vi "SVT UFF58 Get Function References.vi"(0 "file refnum":refnum<k20>, 5 "function type (all functions:0)":T2, 11 "error in (no error)":errorcluster) -> (4 "dup file refnum":refnum<k20>, 6 "function refnums":refnum<k20>[](array[refnum]), 8 "function types":T1[](array[typedef]), 10 "number of functions":i32, 15 "error out":errorcluster)   [LabVIEW 2017, in "SoundVib_UFF58.lvlib"]
doc: "Retrieves the function references and the function types of all the functions specified by <B>function type</B> that are present in the UFF58 (universal file format) file specified by <B>file refnum</B>."
uses:
  <vilib>/addons/Sound and Vibration/svt_UFF58/SoundVib_UFF58.lvlib
  <vilib>/addons/Sound and Vibration/svt_UFF58/subVIs/sv_UFF58 Get FunctionType.ctl
  <vilib>/addons/Sound and Vibration/svt_UFF58/subVIs/sv_FunctionType.ctl
  <vilib>/Platform/storage/Storage.llb/Get Property (Storage Refnums).vi
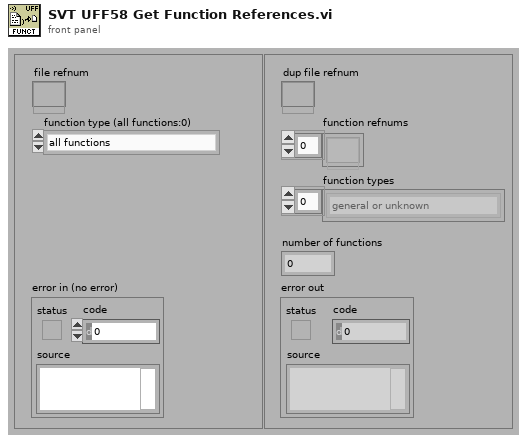
[diagram p1: front panel]
types:
  T1 = typedef "SoundVib_UFF58.lvlib/sv_FunctionType.ctl" = enum16{"general or unknown", "time response", "auto spectrum", "cross spectrum", "frequency response function", "transmissibility", "coherence", "auto correlation", "cross correlation", "power spectral density (PSD)", "energy spectral density (ESD)", "probability density function", "spectrum", "cumulative frequency distribution", "peaks valley", "stress/cycles", "strain/cycles", "orbit", "mode indicator function", "force pattern", "partial power", "partial coherence", "eigenvalue", "eigenvector", "shock response spectrum", "finite impulse response filter", "multiple coherence", "order function", "phase compensation"}
  T2 = typedef "SoundVib_UFF58.lvlib/sv_UFF58 Get FunctionType.ctl" = enum16{"all functions", "all time waveforms", "all spectra (real)", "all spectra (complex)", "general or unknown", "time response", "auto spectrum", "cross spectrum", "frequency response function", "transmissibility", "coherence", "auto correlation", "cross correlation", "power spectral density (PSD)", "energy spectral density (ESD)", "probability density function", "spectrum", "cumulative frequency distribution", "peaks valley", "stress/cycles", "strain/cycles", "orbit", "mode indicator function", "force pattern", "partial power", "partial coherence", "eigenvalue", "eigenvector", "shock response spectrum", "finite impulse response filter", "multiple coherence", "order function"}
  T3 = typedef "SoundVib_UFF58.lvlib/sv_UFF58 DOF.ctl" = cluster{"function type":T1, "function ID number":i32, "version number":i32, "load case ID number":i32, "response entity name":string, "response node":i32, "response direction":T4, "reference entity name":string, "reference node":i32, "reference direction":T4}
  T4 = typedef "SoundVib_UFF58.lvlib/sv_UFF58 Response Direction.ctl" = i32
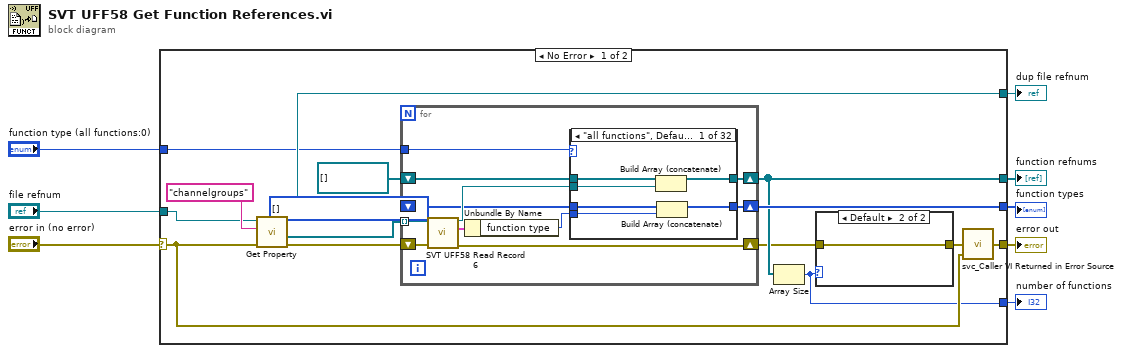
[diagram p0: block diagram]
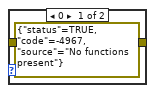
[diagram p2: hidden frame]
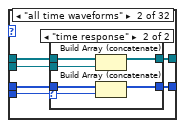
[diagram p3: hidden frame]
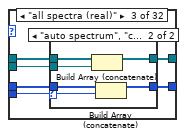
[diagram p5: hidden frame]
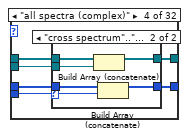
[diagram p7: hidden frame]
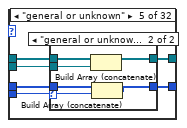
[diagram p9: hidden frame]
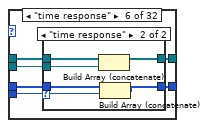
[diagram p11: hidden frame]
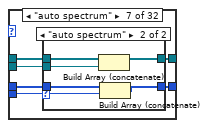
[diagram p13: hidden frame]
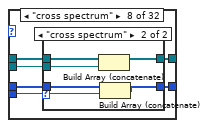
[diagram p15: hidden frame]
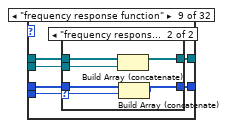
[diagram p17: hidden frame]
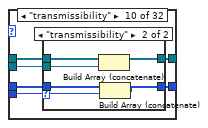
[diagram p19: hidden frame]
diagram:
  n1 = case shown="No Error" "error in (no error)" {
    selector: "error in (no error)" -> [w18 w477]
    tunnel: "file refnum" -> [w22 w478]
    tunnel: [w21 w478] -> w2
    tunnel: [w11 _] -> w7
    tunnel: [w12 _] -> w6
    tunnel: [w14 _] -> w5
    tunnel: [w19 w477] -> w4
    tunnel: "function type (all functions:0)" -> [w15 _]
    frame No Error {
      w16 = T1[] [] items=["general or unknown", "time response", "auto spectrum", "cross spectrum", "frequency response function", "transmissibility", "coherence", "auto correlation", "cross correlation", "power spectral density (PSD)", "energy spectral density (ESD)", "probability density function", "spectrum", "cumulative frequency distribution", "peaks valley", "stress/cycles", "strain/cycles", "orbit", "mode indicator function", "force pattern", "partial power", "partial coherence", "eigenvalue", "eigenvector", "shock response spectrum", "finite impulse response filter", "multiple coherence", "order function", "phase compensation"]
      n2 = call-poly <vilib>:"Get Property.vi"("error in (no error)"=w18, "Property name"="channelgroups", "storage refnum"=w22) -> ("error out"=w20:errorcluster, "Value"=w17:refnum<k20>[], "storage refnum out"=w21:refnum<k20>)  [unwired: 6 in]
      n3 = for {
        tunnel: w17 -> [w33] mode=indexing
        shift-right: [w34] -> w10
        shift-left: w20 -> [w35]
        shift-right: [w26] -> w12
        shift-left: refnum<k20>[] [] -> [w27]
        tunnel: w15 -> [w32]
        shift-right: [w30] -> w14
        shift-left: w16 -> [w28]
        n4 = call <vilib>:"SVT UFF58 Read Record 6.vi"("function refnum"=w33, "error in (no error)"=w35) -> ("dup function refnum"=w29:refnum<k20>, "DOF identification"=w36:T3, "error out"=w34:errorcluster)  [unwired: 11 in]
        n5 = Unbundle By Name(w36) -> ("function type"=w31:T1)
        n6 = case shown="\"all functions\", Default" w32 {
          tunnel: w31 -> [w41 w46 w62 w76 w89 w103 w117 w131 w145 w159 w173 w187 w201 w215 w229 w243 w257 w271 w285 w299 w313 w327 w341 w355 w369 w383 w397 w411 w425 w439 w453 w467]
          tunnel: w28 -> [w42 w48 w61 w75 w90 w104 w118 w132 w146 w160 w174 w188 w202 w216 w230 w244 w258 w272 w286 w300 w314 w328 w342 w356 w370 w384 w398 w412 w426 w440 w454 w468]
          tunnel: [w40 w47 w60 w74 w88 w102 w116 w130 w144 w158 w172 w186 w200 w214 w228 w242 w256 w270 w284 w298 w312 w326 w340 w354 w368 w382 w396 w410 w424 w438 w452 w466] -> w30
          tunnel: w29 -> [w38 w44 w58 w72 w85 w99 w113 w127 w141 w155 w169 w183 w197 w211 w225 w239 w253 w267 w281 w295 w309 w323 w337 w351 w365 w379 w393 w407 w421 w435 w449 w463]
          tunnel: w27 -> [w39 w45 w59 w73 w87 w101 w115 w129 w143 w157 w171 w185 w199 w213 w227 w241 w255 w269 w283 w297 w311 w325 w339 w353 w367 w381 w395 w409 w423 w437 w451 w465]
          tunnel: [w37 w43 w57 w71 w86 w100 w114 w128 w142 w156 w170 w184 w198 w212 w226 w240 w254 w268 w282 w296 w310 w324 w338 w352 w366 w380 w394 w408 w422 w436 w450 w464] -> w26
          frame "all functions", Default {
            n7 = Build Array (concatenate)(w39, w38) -> (w37:refnum<k20>[])
            n8 = Build Array (concatenate)(w42, w41) -> (w40:T1[])
          }
          frame "all time waveforms" {
            n9 = case shown="\"time response\"" w46 {
              selector: w46 -> [_ w54]
              tunnel: w48 -> [w50 w56]
              tunnel: [w50 w55] -> w47
              tunnel: w45 -> [w49 w53]
              tunnel: w44 -> [_ w52]
              tunnel: [w49 w51] -> w43
              frame Default {
              }
              frame "time response" {
                n10 = Build Array (concatenate)(w53, w52) -> (w51:refnum<k20>[])
                n11 = Build Array (concatenate)(w56, w54) -> (w55:T1[])
              }
            }
          }
          frame "all spectra (real)" {
            n12 = case shown="\"auto spectrum\", \"coherence\", \"power spectral density (PSD)\", \"energy spectral density (ESD)\", \"spectrum\", \"partial power\", \"partial coherence\", \"shock response spectrum\"" w62 {
              selector: w62 -> [_ w68]
              tunnel: w61 -> [w64 w70]
              tunnel: [w64 w69] -> w60
              tunnel: w59 -> [w63 w67]
              tunnel: w58 -> [_ w66]
              tunnel: [w63 w65] -> w57
              frame Default {
              }
              frame "auto spectrum", "coherence", "power spectral density (PSD)", "energy spectral density (ESD)", "spectrum", "partial power", "partial coherence", "shock response spectrum" {
                n13 = Build Array (concatenate)(w67, w66) -> (w65:refnum<k20>[])
                n14 = Build Array (concatenate)(w70, w68) -> (w69:T1[])
              }
            }
          }
          frame "all spectra (complex)" {
            n15 = case shown="\"cross spectrum\"..\"transmissibility\", \"peaks valley\"..\"orbit\"" w76 {
              selector: w76 -> [_ w82]
              tunnel: w75 -> [w78 w84]
              tunnel: [w78 w83] -> w74
              tunnel: w73 -> [w77 w81]
              tunnel: w72 -> [_ w80]
              tunnel: [w77 w79] -> w71
              frame Default {
              }
              frame "cross spectrum".."transmissibility", "peaks valley".."orbit" {
                n16 = Build Array (concatenate)(w81, w80) -> (w79:refnum<k20>[])
                n17 = Build Array (concatenate)(w84, w82) -> (w83:T1[])
              }
            }
          }
          frame "general or unknown" {
            n18 = case shown="\"general or unknown\"" w89 {
              selector: w89 -> [_ w97]
              tunnel: w90 -> [w92 w98]
              tunnel: [w92 w96] -> w88
              tunnel: w87 -> [w91 w95]
              tunnel: [w91 w94] -> w86
              tunnel: w85 -> [_ w93]
              frame Default {
              }
              frame "general or unknown" {
                n19 = Build Array (concatenate)(w95, w93) -> (w94:refnum<k20>[])
                n20 = Build Array (concatenate)(w98, w97) -> (w96:T1[])
              }
            }
          }
          frame "time response" {
            n21 = case shown="\"time response\"" w103 {
              selector: w103 -> [_ w111]
              tunnel: w104 -> [w106 w112]
              tunnel: [w106 w110] -> w102
              tunnel: w101 -> [w105 w109]
              tunnel: [w105 w108] -> w100
              tunnel: w99 -> [_ w107]
              frame Default {
              }
              frame "time response" {
                n22 = Build Array (concatenate)(w109, w107) -> (w108:refnum<k20>[])
                n23 = Build Array (concatenate)(w112, w111) -> (w110:T1[])
              }
            }
          }
          frame "auto spectrum" {
            n24 = case shown="\"auto spectrum\"" w117 {
              selector: w117 -> [_ w125]
              tunnel: w118 -> [w120 w126]
              tunnel: [w120 w124] -> w116
              tunnel: w115 -> [w119 w123]
              tunnel: [w119 w122] -> w114
              tunnel: w113 -> [_ w121]
              frame Default {
              }
              frame "auto spectrum" {
                n25 = Build Array (concatenate)(w123, w121) -> (w122:refnum<k20>[])
                n26 = Build Array (concatenate)(w126, w125) -> (w124:T1[])
              }
            }
          }
          frame "cross spectrum" {
            n27 = case shown="\"cross spectrum\"" w131 {
              selector: w131 -> [_ w139]
              tunnel: w132 -> [w134 w140]
              tunnel: [w134 w138] -> w130
              tunnel: w129 -> [w133 w137]
              tunnel: [w133 w136] -> w128
              tunnel: w127 -> [_ w135]
              frame Default {
              }
              frame "cross spectrum" {
                n28 = Build Array (concatenate)(w137, w135) -> (w136:refnum<k20>[])
                n29 = Build Array (concatenate)(w140, w139) -> (w138:T1[])
              }
            }
          }
          frame "frequency response function" {
            n30 = case shown="\"frequency response function\"" w145 {
              selector: w145 -> [_ w153]
              tunnel: w146 -> [w148 w154]
              tunnel: [w148 w152] -> w144
              tunnel: w143 -> [w147 w151]
              tunnel: [w147 w150] -> w142
              tunnel: w141 -> [_ w149]
              frame Default {
              }
              frame "frequency response function" {
                n31 = Build Array (concatenate)(w151, w149) -> (w150:refnum<k20>[])
                n32 = Build Array (concatenate)(w154, w153) -> (w152:T1[])
              }
            }
          }
          frame "transmissibility" {
            n33 = case shown="\"transmissibility\"" w159 {
              selector: w159 -> [_ w167]
              tunnel: w160 -> [w162 w168]
              tunnel: [w162 w166] -> w158
              tunnel: w157 -> [w161 w165]
              tunnel: [w161 w164] -> w156
              tunnel: w155 -> [_ w163]
              frame Default {
              }
              frame "transmissibility" {
                n34 = Build Array (concatenate)(w165, w163) -> (w164:refnum<k20>[])
                n35 = Build Array (concatenate)(w168, w167) -> (w166:T1[])
              }
            }
          }
          frame "coherence" {
            n36 = case shown="\"coherence\"" w173 {
              selector: w173 -> [_ w181]
              tunnel: w174 -> [w176 w182]
              tunnel: [w176 w180] -> w172
              tunnel: w171 -> [w175 w179]
              tunnel: [w175 w178] -> w170
              tunnel: w169 -> [_ w177]
              frame Default {
              }
              frame "coherence" {
                n37 = Build Array (concatenate)(w179, w177) -> (w178:refnum<k20>[])
                n38 = Build Array (concatenate)(w182, w181) -> (w180:T1[])
              }
            }
          }
          frame "auto correlation" {
            n39 = case shown="\"auto correlation\"" w187 {
              selector: w187 -> [_ w195]
              tunnel: w188 -> [w190 w196]
              tunnel: [w190 w194] -> w186
              tunnel: w185 -> [w189 w193]
              tunnel: [w189 w192] -> w184
              tunnel: w183 -> [_ w191]
              frame Default {
              }
              frame "auto correlation" {
                n40 = Build Array (concatenate)(w193, w191) -> (w192:refnum<k20>[])
                n41 = Build Array (concatenate)(w196, w195) -> (w194:T1[])
              }
            }
          }
          frame "cross correlation" {
            n42 = case shown="\"cross correlation\"" w201 {
              selector: w201 -> [_ w209]
              tunnel: w202 -> [w204 w210]
              tunnel: [w204 w208] -> w200
              tunnel: w199 -> [w203 w207]
              tunnel: [w203 w206] -> w198
              tunnel: w197 -> [_ w205]
              frame Default {
              }
              frame "cross correlation" {
                n43 = Build Array (concatenate)(w207, w205) -> (w206:refnum<k20>[])
                n44 = Build Array (concatenate)(w210, w209) -> (w208:T1[])
              }
            }
          }
          frame "power spectral density (PSD)" {
            n45 = case shown="\"power spectral density (PSD)\"" w215 {
              selector: w215 -> [_ w223]
              tunnel: w216 -> [w218 w224]
              tunnel: [w218 w222] -> w214
              tunnel: w213 -> [w217 w221]
              tunnel: [w217 w220] -> w212
              tunnel: w211 -> [_ w219]
              frame Default {
              }
              frame "power spectral density (PSD)" {
                n46 = Build Array (concatenate)(w221, w219) -> (w220:refnum<k20>[])
                n47 = Build Array (concatenate)(w224, w223) -> (w222:T1[])
              }
            }
          }
          frame "energy spectral density (ESD)" {
            n48 = case shown="\"energy spectral density (ESD)\"" w229 {
              selector: w229 -> [_ w237]
              tunnel: w230 -> [w232 w238]
              tunnel: [w232 w236] -> w228
              tunnel: w227 -> [w231 w235]
              tunnel: [w231 w234] -> w226
              tunnel: w225 -> [_ w233]
              frame Default {
              }
              frame "energy spectral density (ESD)" {
                n49 = Build Array (concatenate)(w235, w233) -> (w234:refnum<k20>[])
                n50 = Build Array (concatenate)(w238, w237) -> (w236:T1[])
              }
            }
          }
          frame "probability density function" {
            n51 = case shown="\"probability density function\"" w243 {
              selector: w243 -> [_ w251]
              tunnel: w244 -> [w246 w252]
              tunnel: [w246 w250] -> w242
              tunnel: w241 -> [w245 w249]
              tunnel: [w245 w248] -> w240
              tunnel: w239 -> [_ w247]
              frame Default {
              }
              frame "probability density function" {
                n52 = Build Array (concatenate)(w249, w247) -> (w248:refnum<k20>[])
                n53 = Build Array (concatenate)(w252, w251) -> (w250:T1[])
              }
            }
          }
          frame "spectrum" {
            n54 = case shown="\"spectrum\"" w257 {
              selector: w257 -> [_ w265]
              tunnel: w258 -> [w260 w266]
              tunnel: [w260 w264] -> w256
              tunnel: w255 -> [w259 w263]
              tunnel: [w259 w262] -> w254
              tunnel: w253 -> [_ w261]
              frame Default {
              }
              frame "spectrum" {
                n55 = Build Array (concatenate)(w263, w261) -> (w262:refnum<k20>[])
                n56 = Build Array (concatenate)(w266, w265) -> (w264:T1[])
              }
            }
          }
          frame "cumulative frequency distribution" {
            n57 = case shown="\"cumulative frequency distribution\"" w271 {
              selector: w271 -> [_ w279]
              tunnel: w272 -> [w274 w280]
              tunnel: [w274 w278] -> w270
              tunnel: w269 -> [w273 w277]
              tunnel: [w273 w276] -> w268
              tunnel: w267 -> [_ w275]
              frame Default {
              }
              frame "cumulative frequency distribution" {
                n58 = Build Array (concatenate)(w277, w275) -> (w276:refnum<k20>[])
                n59 = Build Array (concatenate)(w280, w279) -> (w278:T1[])
              }
            }
          }
          frame "peaks valley" {
            n60 = case shown="\"peaks valley\"" w285 {
              selector: w285 -> [_ w293]
              tunnel: w286 -> [w288 w294]
              tunnel: [w288 w292] -> w284
              tunnel: w283 -> [w287 w291]
              tunnel: [w287 w290] -> w282
              tunnel: w281 -> [_ w289]
              frame Default {
              }
              frame "peaks valley" {
                n61 = Build Array (concatenate)(w291, w289) -> (w290:refnum<k20>[])
                n62 = Build Array (concatenate)(w294, w293) -> (w292:T1[])
              }
            }
          }
          frame "stress/cycles" {
            n63 = case shown="\"stress/cycles\"" w299 {
              selector: w299 -> [_ w307]
              tunnel: w300 -> [w302 w308]
              tunnel: [w302 w306] -> w298
              tunnel: w297 -> [w301 w305]
              tunnel: [w301 w304] -> w296
              tunnel: w295 -> [_ w303]
              frame Default {
              }
              frame "stress/cycles" {
                n64 = Build Array (concatenate)(w305, w303) -> (w304:refnum<k20>[])
                n65 = Build Array (concatenate)(w308, w307) -> (w306:T1[])
              }
            }
          }
          frame "strain/cycles" {
            n66 = case shown="\"strain/cycles\"" w313 {
              selector: w313 -> [_ w321]
              tunnel: w314 -> [w316 w322]
              tunnel: [w316 w320] -> w312
              tunnel: w311 -> [w315 w319]
              tunnel: [w315 w318] -> w310
              tunnel: w309 -> [_ w317]
              frame Default {
              }
              frame "strain/cycles" {
                n67 = Build Array (concatenate)(w319, w317) -> (w318:refnum<k20>[])
                n68 = Build Array (concatenate)(w322, w321) -> (w320:T1[])
              }
            }
          }
          frame "orbit" {
            n69 = case shown="\"orbit\"" w327 {
              selector: w327 -> [_ w335]
              tunnel: w328 -> [w330 w336]
              tunnel: [w330 w334] -> w326
              tunnel: w325 -> [w329 w333]
              tunnel: [w329 w332] -> w324
              tunnel: w323 -> [_ w331]
              frame Default {
              }
              frame "orbit" {
                n70 = Build Array (concatenate)(w333, w331) -> (w332:refnum<k20>[])
                n71 = Build Array (concatenate)(w336, w335) -> (w334:T1[])
              }
            }
          }
          frame "mode indicator function" {
            n72 = case shown="\"mode indicator function\"" w341 {
              selector: w341 -> [_ w349]
              tunnel: w342 -> [w344 w350]
              tunnel: [w344 w348] -> w340
              tunnel: w339 -> [w343 w347]
              tunnel: [w343 w346] -> w338
              tunnel: w337 -> [_ w345]
              frame Default {
              }
              frame "mode indicator function" {
                n73 = Build Array (concatenate)(w347, w345) -> (w346:refnum<k20>[])
                n74 = Build Array (concatenate)(w350, w349) -> (w348:T1[])
              }
            }
          }
          frame "force pattern" {
            n75 = case shown="\"force pattern\"" w355 {
              selector: w355 -> [_ w363]
              tunnel: w356 -> [w358 w364]
              tunnel: [w358 w362] -> w354
              tunnel: w353 -> [w357 w361]
              tunnel: [w357 w360] -> w352
              tunnel: w351 -> [_ w359]
              frame Default {
              }
              frame "force pattern" {
                n76 = Build Array (concatenate)(w361, w359) -> (w360:refnum<k20>[])
                n77 = Build Array (concatenate)(w364, w363) -> (w362:T1[])
              }
            }
          }
          frame "partial power" {
            n78 = case shown="\"partial power\"" w369 {
              selector: w369 -> [_ w377]
              tunnel: w370 -> [w372 w378]
              tunnel: [w372 w376] -> w368
              tunnel: w367 -> [w371 w375]
              tunnel: [w371 w374] -> w366
              tunnel: w365 -> [_ w373]
              frame Default {
              }
              frame "partial power" {
                n79 = Build Array (concatenate)(w375, w373) -> (w374:refnum<k20>[])
                n80 = Build Array (concatenate)(w378, w377) -> (w376:T1[])
              }
            }
          }
          frame "partial coherence" {
            n81 = case shown="\"partial coherence\"" w383 {
              selector: w383 -> [_ w391]
              tunnel: w384 -> [w386 w392]
              tunnel: [w386 w390] -> w382
              tunnel: w381 -> [w385 w389]
              tunnel: [w385 w388] -> w380
              tunnel: w379 -> [_ w387]
              frame Default {
              }
              frame "partial coherence" {
                n82 = Build Array (concatenate)(w389, w387) -> (w388:refnum<k20>[])
                n83 = Build Array (concatenate)(w392, w391) -> (w390:T1[])
              }
            }
          }
          frame "eigenvalue" {
            n84 = case shown="\"eigenvalue\"" w397 {
              selector: w397 -> [_ w405]
              tunnel: w398 -> [w400 w406]
              tunnel: [w400 w404] -> w396
              tunnel: w395 -> [w399 w403]
              tunnel: [w399 w402] -> w394
              tunnel: w393 -> [_ w401]
              frame Default {
              }
              frame "eigenvalue" {
                n85 = Build Array (concatenate)(w403, w401) -> (w402:refnum<k20>[])
                n86 = Build Array (concatenate)(w406, w405) -> (w404:T1[])
              }
            }
          }
          frame "eigenvector" {
            n87 = case shown="\"eigenvector\"" w411 {
              selector: w411 -> [_ w419]
              tunnel: w412 -> [w414 w420]
              tunnel: [w414 w418] -> w410
              tunnel: w409 -> [w413 w417]
              tunnel: [w413 w416] -> w408
              tunnel: w407 -> [_ w415]
              frame Default {
              }
              frame "eigenvector" {
                n88 = Build Array (concatenate)(w417, w415) -> (w416:refnum<k20>[])
                n89 = Build Array (concatenate)(w420, w419) -> (w418:T1[])
              }
            }
          }
          frame "shock response spectrum" {
            n90 = case shown="\"shock response spectrum\"" w425 {
              selector: w425 -> [_ w433]
              tunnel: w426 -> [w428 w434]
              tunnel: [w428 w432] -> w424
              tunnel: w423 -> [w427 w431]
              tunnel: [w427 w430] -> w422
              tunnel: w421 -> [_ w429]
              frame Default {
              }
              frame "shock response spectrum" {
                n91 = Build Array (concatenate)(w431, w429) -> (w430:refnum<k20>[])
                n92 = Build Array (concatenate)(w434, w433) -> (w432:T1[])
              }
            }
          }
          frame "finite impulse response filter" {
            n93 = case shown="\"finite impulse response filter\"" w439 {
              selector: w439 -> [_ w447]
              tunnel: w440 -> [w442 w448]
              tunnel: [w442 w446] -> w438
              tunnel: w437 -> [w441 w445]
              tunnel: [w441 w444] -> w436
              tunnel: w435 -> [_ w443]
              frame Default {
              }
              frame "finite impulse response filter" {
                n94 = Build Array (concatenate)(w445, w443) -> (w444:refnum<k20>[])
                n95 = Build Array (concatenate)(w448, w447) -> (w446:T1[])
              }
            }
          }
          frame "multiple coherence" {
            n96 = case shown="\"multiple coherence\"" w453 {
              selector: w453 -> [_ w461]
              tunnel: w454 -> [w456 w462]
              tunnel: [w456 w460] -> w452
              tunnel: w451 -> [w455 w459]
              tunnel: [w455 w458] -> w450
              tunnel: w449 -> [_ w457]
              frame Default {
              }
              frame "multiple coherence" {
                n97 = Build Array (concatenate)(w459, w457) -> (w458:refnum<k20>[])
                n98 = Build Array (concatenate)(w462, w461) -> (w460:T1[])
              }
            }
          }
          frame "order function" {
            n99 = case shown="\"order function\"" w467 {
              selector: w467 -> [_ w475]
              tunnel: w468 -> [w470 w476]
              tunnel: [w470 w474] -> w466
              tunnel: w465 -> [w469 w473]
              tunnel: [w469 w472] -> w464
              tunnel: w463 -> [_ w471]
              frame Default {
              }
              frame "order function" {
                n100 = Build Array (concatenate)(w473, w471) -> (w472:refnum<k20>[])
                n101 = Build Array (concatenate)(w476, w475) -> (w474:T1[])
              }
            }
          }
        }
      }
      n102 = Array Size(array=w12) -> (size(s)=w11:i32)
      n103 = case shown="Default" w11 {
        tunnel: w10 -> [_ w25]
        tunnel: [errorcluster {"status"=TRUE, "code"=-4967, "source"="No functions present"} ("error out") w25] -> w9
        frame 0 {
        }
        frame Default {
        }
      }
      n104 = call <vilib>:"svc_Caller VI Returned in Error Source.vi"("warning input to caller"=w18, "error in (no error)"=w9) -> ("error out"=w19:errorcluster)  [unwired: 3 in]
    }
    frame Error {
    }
  }
  "error out" <- w4
  "function refnums" <- w6
  "number of functions" <- w7
  "dup file refnum" <- w2
  "function types" <- w5
